vi "parseDataI8.vi"(8 "error in (no error)":errorcluster, 11 "FrameParser in":refnum<class "FrameParser.lvclass">) -> (0 "error out":errorcluster, 2 "Data":i8, 3 "FrameParser out":refnum<class "FrameParser.lvclass">)   [LabVIEW 2015, in "RTModbus.lvlib" / "FrameParser.lvclass"]
uses:
  FrameParser.lvclass
  FrameParser.lvclass/FrameParser.ctl
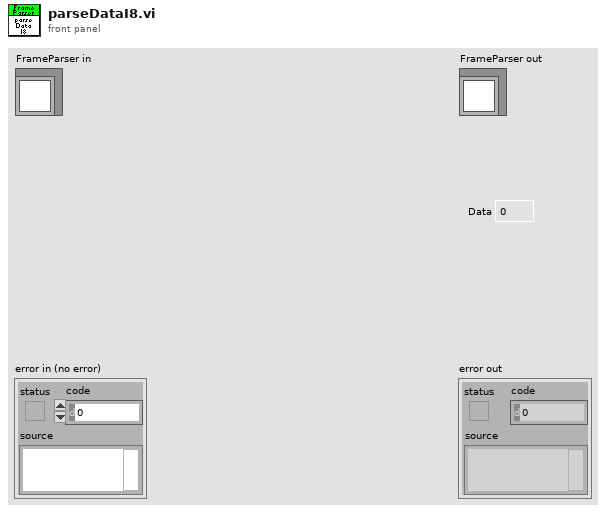
[diagram p1: front panel]
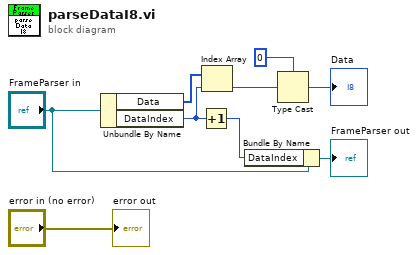
[diagram p0: block diagram]
diagram:
  n1 = Unbundle By Name("FrameParser in") -> ("Data"=w9:u8[], "DataIndex"=w3:i32)
  n2 = Increment(x=w3) -> (x+1=w4:i32)
  n3 = Index Array(array=w9, index=w3) -> (element=w7:u8)
  n4 = Bundle By Name(cluster="FrameParser in", "DataIndex"=w4) -> (→"FrameParser out":refnum<class "FrameParser.lvclass">)
  n5 = Type Cast(type=i8 0 ("Data"), x=w7) -> (*(type *) &x=→"Data":i8)
  "error out" <- "error in (no error)"
